vi "G# - DebugServer.vi"() -> ()   [LabVIEW 2017]
doc: "Debug Server\nThis examples shows how the debug server works. The debug server is used to remotely debug G# applications.\n\nThis applications could be an LabVIEW RT system, LabVIEW web services, LabVIEW build executables and also just another application instance.\n\nIn this example a temporary project is launched (causing a new application instance) and the G# Debugger is launched from this project. When the debugger launches, press \"Connect\" and enter \"localhost\" as the target address. You now see the objects being created and destroyed on the remote target. Notice also the debugger trace and the user events that are being logged."
uses:
  MyRemoteClass_class/MyRemoteClass.lvclass
  C:/Program Files/National Instruments/LabVIEW 2017/vi.lib/addons/_AddQ/G#Object/G#Object.lvclass
  <vilib>/addons/_AddQ/G#DebugServer/G#DebugServer.lvclass
  <vilib>/addons/_AddQ/G#Object/G#Object.lvclass
  <vilib>/addons/_AddQ/G#Debugger/G#Debugger.lvlib
panel:
  in  "stop":bool
  out "error out":errorcluster
  # "Debug Server\nThis examples shows how the debug server works. The debug server is used to remotely debug G# applications.\n\nThis applications could be an LabVIEW RT system, LabVIEW web services, LabVIEW build executables and also just another application instance.\n\nIn this example a temporary project is launched (causing a new application instance) and the G# Debugger is launched from this project. When the debugger launches, press \"Connect\" and enter \"localhost\" as the target address. You now see the objects being created and destroyed on the remote target. Notice also the debugger trace and the user events that are being logged."
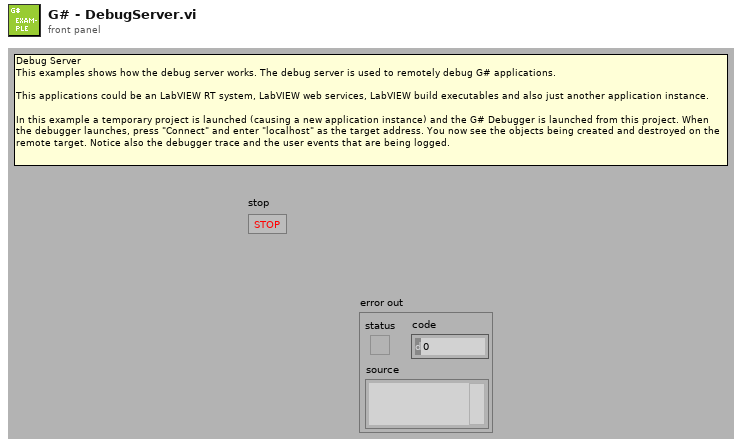
[diagram p1: front panel]
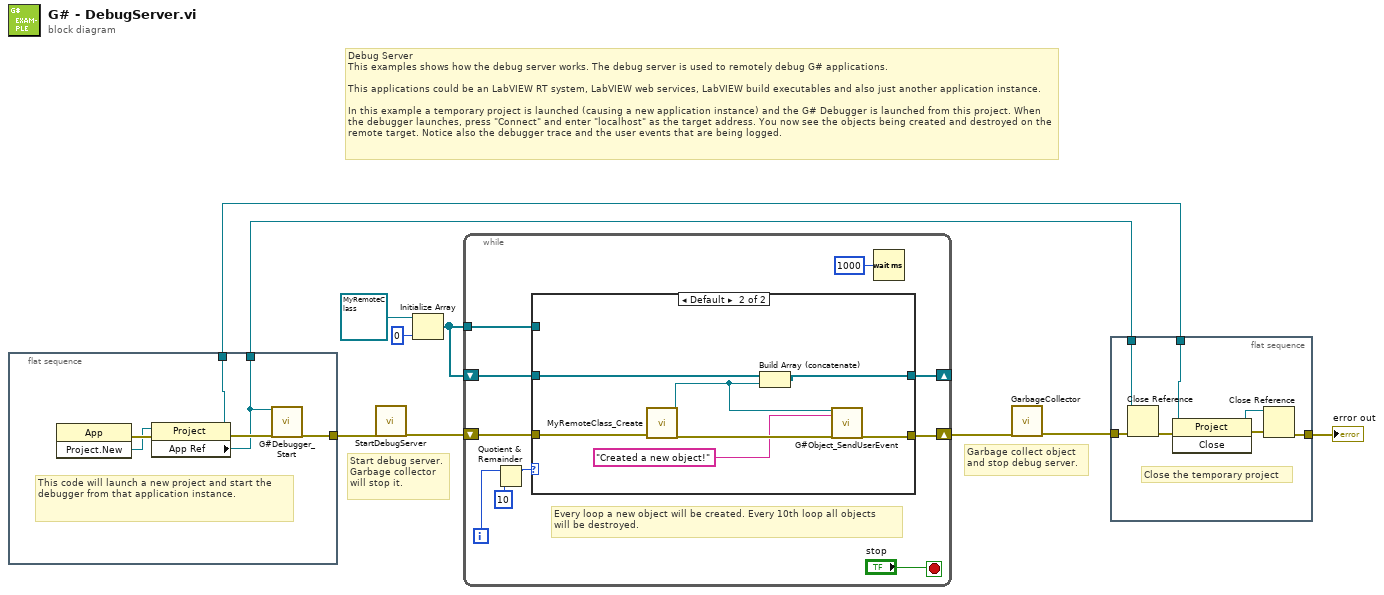
[diagram p0: block diagram]
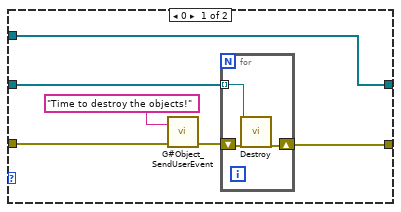
[diagram p2: hidden frame]
diagram:
  # "Garbage collect object\nand stop debug server."
  # "Start debug server.\nGarbage collector\nwill stop it."
  # "Debug Server\nThis examples shows how the debug server works. The debug server is used to remotely debug G# applications.\n\nThis applications could be an LabVIEW RT system, LabVIEW web services, LabVIEW build executables and also just another application instance.\n\nIn this example a temporary project is launched (causing a new application instance) and the G# Debugger is launched from this project. When the debugger launches, press \"Connect\" and enter \"localhost\" as the target address. You now see the objects being created and destroyed on the remote target. Notice also the debugger trace and the user events that are being logged."
  n1 = flat-sequence {
    tunnel: [w13] -> w5
    tunnel: [w12] -> w3
    tunnel: [w11] -> w2
    frame #0 {
      # "This code will launch a new project and start the\ndebugger from that application instance."
      n2 = invoke class="App" method="Project.New"() -> (error out=w16:errorcluster, "Project:New"=w15:refnum<vi>)  [unwired: 3 in, 1 out]
      n3 = property class="Project"(reference=w15, error in=w16) -> (reference out=w11:refnum<vi>, error out=w14:errorcluster, "App Ref"=w12:refnum<vi>)
      n4 = call <vilib>:"G#Debugger_Start.vi"("application reference"=w12, "error in (no error)"=w14) -> ("error out"=w13:errorcluster)  [unwired: 17 in]
    }
  }
  n5 = call <vilib>:"StartDebugServer.vi"("error in (no error)"=w5) -> ("error out"=w10:errorcluster)  [unwired: 18 in]
  n6 = Initialize Array(refnum<class "MyRemoteClass.lvclass"> refnum ("reference out"), 0 ("dimension size")) -> (w7:refnum<class "MyRemoteClass.lvclass">[])
  n7 = while {
    shift-right: [w20] -> _
    shift-left: w7 -> [w21]
    shift-right: [w18] -> w6
    shift-left: w10 -> [w25]
    tunnel: w7 -> [w19]
    i -> [w24]
    stop <- "stop" stop-if-true
    # "Every loop a new object will be created. Every 10th loop all objects\nwill be destroyed."
    n8 = Quotient & Remainder(x=w24, y=10) -> (x-y*floor(x/y)=w22:i32)  [unwired: 1 out]
    n9 = case shown="Default" w22 {
      tunnel: w25 -> [w29 w42]
      tunnel: w21 -> [w32 w41]
      tunnel: [w31 w40] -> w20
      tunnel: w19 -> [w31 _]
      tunnel: [w30 w38] -> w18
      frame 0 {
        n10 = call <vilib>:"G#Object_SendUserEvent.vi"("text"="Time to destroy the objects!", "error in (no error)"=w29) -> ("error out"=w28:errorcluster)  [unwired: 16 in, 1 out]
        n11 = for {
          shift-right: [w33] -> w30
          shift-left: w28 -> [w34]
          tunnel: w32 -> [w35] mode=indexing
          n12 = call-dynamic "Destroy.vi"("reference in"=w35, "error in (no error)"=w34) -> ("error out"=w33:errorcluster)  [unwired: 16 in, 1 out]
        }
      }
      frame Default {
        n13 = call "MyRemoteClass_Create.vi"("error in (no error)"=w42) -> ("reference out"=w37:refnum<class "MyRemoteClass.lvclass">, "error out"=w39:errorcluster)  [unwired: 17 in]
        n14 = Build Array (concatenate)(w41, w37) -> (w40:refnum<class "MyRemoteClass.lvclass">[])
        n15 = call <vilib>:"G#Object_SendUserEvent.vi"("refererence in"=w37, "text"="Created a new object!", "error in (no error)"=w39) -> ("error out"=w38:errorcluster)  [unwired: 15 in, 1 out]
      }
    }
    n16 = Wait (ms)(milliseconds to wait=u32 1000) -> ()  [unwired: 1 out]
  }
  n17 = call <vilib>:"GarbageCollector.vi"("error in (no error)"=w6) -> ("error out"=w4:errorcluster)  [unwired: 16 in, 2 out]
  n18 = flat-sequence {
    tunnel: w4 -> [w49]
    tunnel: w3 -> [w48]
    tunnel: w2 -> [w46]
    tunnel: [w43] -> w1
    frame #0 {
      # "Close the temporary project"
      n19 = Close Reference(reference=w48, error in (no error)=w49) -> (error out=w47:errorcluster)
      n20 = invoke class="Project" method="Close"(reference=w46, error in=w47) -> (reference out=w44:refnum<vi>, error out=w45:errorcluster)  [unwired: 1 in, 1 out]
      n21 = Close Reference(reference=w44, error in (no error)=w45) -> (error out=w43:errorcluster)
    }
  }
  "error out" <- w1
